vi "Launch.vi"() -> ()   [LabVIEW 2021, in "CIFCorePlugin.lvclass"]
uses:
  CIFCorePlugin.lvclass
  CIFCorePlugin.lvclass/CIFCorePlugin.ctl
panel:
  in  "Plugin Name":string="Plugin Name Here"
  in  "host ip":string="localhost"
  in  "port":u16=1256
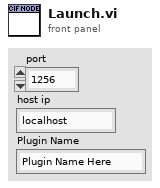
[diagram p1: front panel]
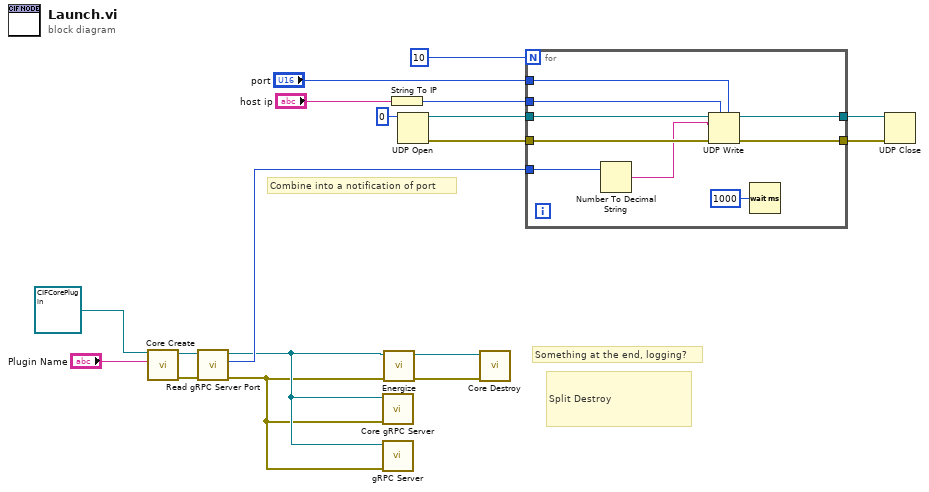
[diagram p0: block diagram]
diagram:
  # "Split Destroy"
  # "Combine into a notification of port"
  # "Something at the end, logging?"
  n1 = call "Core Create.vi"("Plugin Name"="Plugin Name", "CIFTemplateNode in"=refnum<class "CIFCorePlugin.lvclass"> refnum ("CIFCorePlugin.lvclass")) -> ("error out"=w1:errorcluster, "CIFTemplateNode out"=w2:refnum<class "CIFCorePlugin.lvclass">)  [unwired: 8 in]
  n2 = call "Read gRPC Server Port.vi"("error in (no error)"=w1, "CIFTemplateNode in"=w2) -> ("error out"=w3:errorcluster, "gRPC Server Port"=w9:i32, "CIFTemplateNode out"=w4:refnum<class "CIFCorePlugin.lvclass">)  [unwired: 7 in]
  n3 = call "Core gRPC Server.vi"("error in (no error)"=w3, "CIFTemplateNode in"=w4) -> ()  [unwired: 8 in, 2 out]
  n4 = call-dynamic "gRPC Server.vi"("error in (no error)"=w3, "CIFTemplateNode in"=w4) -> ()  [unwired: 8 in, 2 out]
  n5 = call "Energize.vi"("error in (no error)"=w3, "CIFCorePlugin in"=w4) -> ("error out"=w6:errorcluster, "CIFCorePlugin out"=w7:refnum<class "CIFCorePlugin.lvclass">)  [unwired: 8 in]
  n6 = String To IP(1:"host ip") -> (0:w14:u32)
  n7 = UDP Open(11:u16 0 ("port")) -> (port=w17:refnum<k16>, 0:w16:errorcluster)  [unwired: 4 in, 1 out]
  n8 = call "Core Destroy.vi"("error in (no error)"=w6, "CIFTemplateNode in"=w7) -> ()  [unwired: 8 in, 2 out]
  n9 = for {
    N: 10 -> [_]
    tunnel: w17 -> [w27]
    tunnel: w16 -> [w26]
    tunnel: "port" -> [w25]
    tunnel: w14 -> [w24]
    tunnel: [w21] -> w11
    tunnel: [w20] -> w10
    tunnel: w9 -> [w19]
    n10 = Number To Decimal String(number=w19) -> (decimal integer string=w22:string)  [unwired: 1 in]
    n11 = UDP Write(address=w24, port or service name=w25, connection ID=w27, data in=w22, 8:w26) -> (error out=w20:errorcluster, 3:w21:refnum<k16>)  [unwired: 1 in]
    n12 = Wait (ms)(milliseconds to wait=u32 1000) -> ()  [unwired: 1 out]
  }
  n13 = UDP Close(connection ID=w11, 8:w10) -> ()  [unwired: 2 out]
